vi "ReadWrite Binary.vi"() -> ()   [LabVIEW 2014]
panel:
  in  "Data type":enum16{"U8", "I16"}(ring)
  in  "Tab Control":enum32{"Write", "Read"}(tab)
  in  "Array":i16[][](array[numeric])
  out "data":i32[](array[numeric])
  in  "T = AddNewData\nF = if exist, OverWrite or CreateNew":bool
  in  "Read or Write Path":path
  in  "T = Save\nF = Read":bool
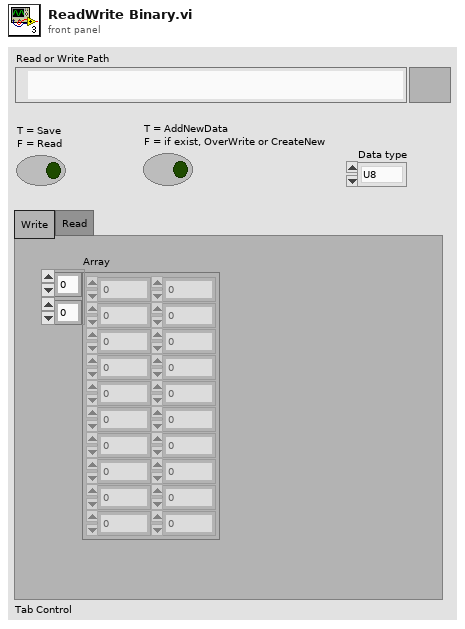
[diagram p1: front panel]
types:
  T1 = enum16{"big-endian, network order", "native, host order", "little-endian"}
  T2 = enum16{"open", "replace", "create", "open or create", "replace or create", "replace or create with confirmation"}
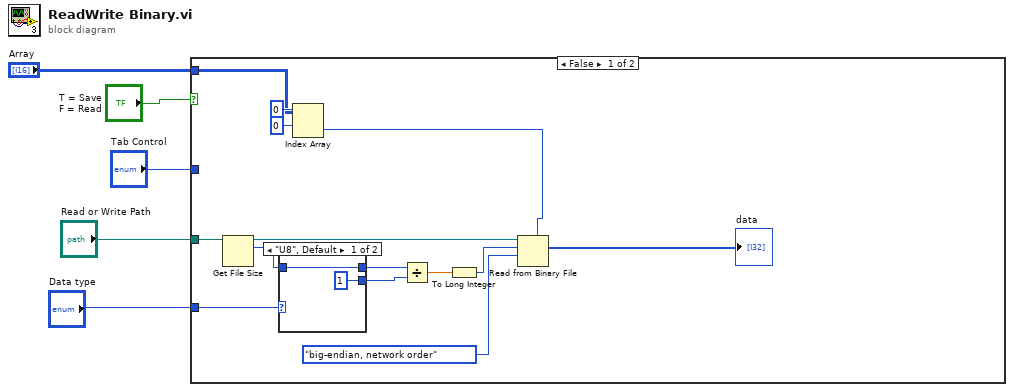
[diagram p0: block diagram]
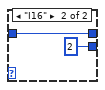
[diagram p2: hidden frame]
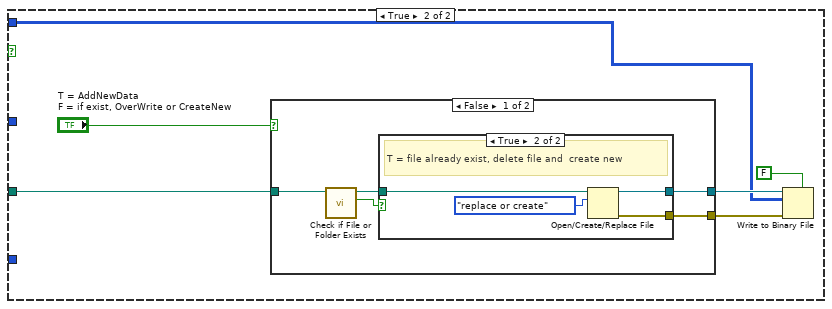
[diagram p3: hidden frame]
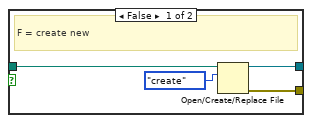
[diagram p4: hidden frame]
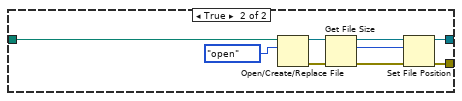
[diagram p5: hidden frame]
diagram:
  n1 = case shown="False" "T = Save\nF = Read" {
    tunnel: "Read or Write Path" -> [w17 w26]
    tunnel: "Tab Control" -> [_ _]
    tunnel: "Array" -> [w8 w24]
    tunnel: "Data type" -> [w6 _]
    frame False {
      n2 = Get File Size(file=w17) -> (refnum out=w16:refnum<file>, size (in bytes)=w14:i64)  [unwired: 1 in, 1 out]
      n3 = case shown="\"U8\", Default" w6 {
        tunnel: [u8 1 i16 2] -> w11
        tunnel: [w21 w22] -> w15
        tunnel: w14 -> [w21 w22]
        frame "U8", Default {
        }
        frame "I16" {
        }
      }
      n4 = Index Array(array=w8, index (row)=0, index (col)=0 ("disabled index (col)")) -> (element=w7:i16)
      n5 = Divide(x=w15, y=w11) -> (x/y=w13:dbl)
      n6 = To Long Integer(number=w13) -> (32bit integer=w12:i32)
      n7 = Read from Binary File(5:w7, 9:T1."big-endian, network order" ("byte order (0:big-endian, network order)"), 10:w12, 11:w16) -> (2:→"data":i16[])  [unwired: 2 in, 3 out]
    }
    frame True {
      n8 = case shown="False" "T = AddNewData\nF = if exist, OverWrite or CreateNew" {
        tunnel: [w31 w50] -> w28
        tunnel: w26 -> [w34 w46]
        tunnel: [w30 w47] -> w25
        frame False {
          n9 = call <vilib>:"Check if File or Folder Exists.vi"("path"=w34) -> ("file or folder exists?"=w33:bool, "dup path"=w32:path)  [unwired: 8 in, 1 out]
          n10 = case shown="True" w33 {
            tunnel: w32 -> [w38 w41]
            tunnel: [w37 w40] -> w31
            tunnel: [w35 w39] -> w30
            frame False {
              # "F = create new"
              n11 = Open/Create/Replace File(file path (use dialog)=w38, operation (0:open)=T2."create") -> (refnum out=w37:refnum<file>, error out=w35:errorcluster)  [unwired: 4 in, 1 out]
            }
            frame True {
              # "T = file already exist, delete file and  create new"
              n12 = Open/Create/Replace File(file path (use dialog)=w41, operation (0:open)=T2."replace or create") -> (refnum out=w40:refnum<file>, error out=w39:errorcluster)  [unwired: 4 in, 1 out]
            }
          }
        }
        frame True {
          n13 = Open/Create/Replace File(file path (use dialog)=w46, operation (0:open)=T2."open") -> (refnum out=w44:refnum<file>, error out=w43:errorcluster)  [unwired: 4 in, 1 out]
          n14 = Get File Size(file=w44, error in=w43) -> (refnum out=w51:refnum<file>, size (in bytes)=w49:i64, 0:w48:errorcluster)
          n15 = Set File Position(offset (in bytes) (0)=w49, refnum=w51, error in=w48) -> (refnum out=w50:refnum<file>, error out=w47:errorcluster)  [unwired: 1 in]
        }
      }
      n16 = Write to Binary File(file (use dialog)=w28, data=w24, error in=w25, 5:FALSE ("prepend array or string size? (T)")) -> ()  [unwired: 2 in, 3 out]
    }
  }
